vi "Write Arguments.vi"(8 "error in (no error)":errorcluster, 10 "Arguments":T1, 11 "ParsedData in":refnum<class "ParsedData.lvclass">) -> (0 "error out":errorcluster, 3 "ParsedData out":refnum<class "ParsedData.lvclass">)   [LabVIEW 2022 SP3, in "ArgumentParser.lvlib" / "ParsedData.lvclass"]
uses:
  ParsedData.lvclass
  ParsedData.lvclass/ParsedData.ctl
  _Arguments.ctl
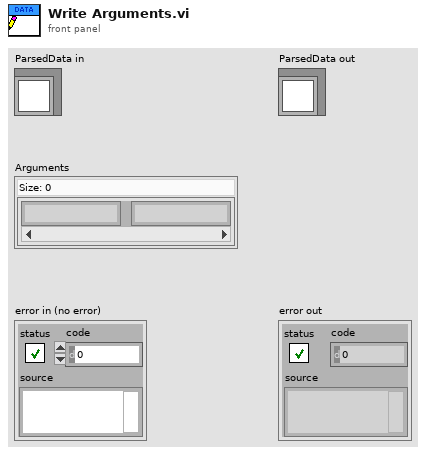
[diagram p1: front panel]
types:
  T1 = typedef "ArgumentParser.lvlib/ParsedData.lvclass/_Arguments.ctl" = map{string, string}
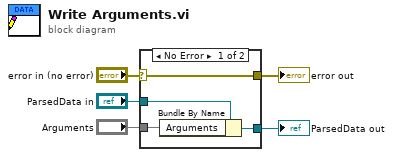
[diagram p0: block diagram]
diagram:
  n1 = case shown="No Error" "error in (no error)" {
    selector: "error in (no error)" -> [w9 w10]
    tunnel: [w9 w10] -> w4
    tunnel: [w7 w11] -> w2
    tunnel: "ParsedData in" -> [w8 w11]
    tunnel: "Arguments" -> [w6 _]
    frame No Error {
      n2 = Bundle By Name(cluster=w8, "Arguments"=w6) -> (w7:refnum<class "ParsedData.lvclass">)
    }
    frame Error {
    }
  }
  "error out" <- w4
  "ParsedData out" <- w2
